vi "Read INI file.vi"(8 "error in (no error)":errorcluster, 11 "App Cluster in":T1) -> (0 "error out":errorcluster, 3 "App Cluster out":T1)   [LabVIEW 2018]
uses:
  type defs/App Cluster.ctl
  <vilib>/Utility/config.llb/Read Key (String).vi
  <vilib>/Utility/config.llb/Read Key (Double).vi
  <vilib>/Utility/config.llb/NI_LVConfig.lvlib
panel:
  out "Parameters":dbl[](array[numeric])
  out "HW":string[](array[string])
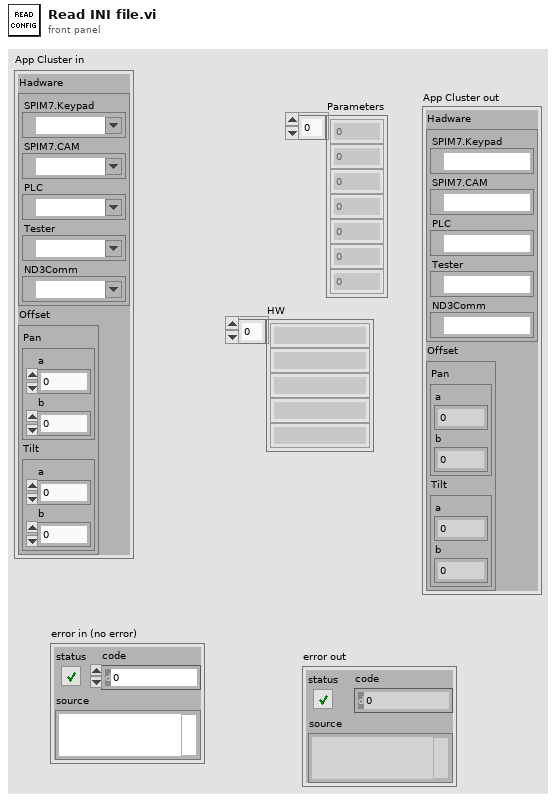
[diagram p1: front panel]
types:
  T1 = typedef "App Cluster.ctl" = cluster{"Hadware":cluster{"SPIM7.Keypad":refnum<visa-resource-name>, "SPIM7.CAM":refnum<visa-resource-name>, "PLC":refnum<visa-resource-name>, "Tester":refnum<visa-resource-name>, "ND3Comm":refnum<visa-resource-name>}, "Offset":cluster{"Pan":cluster{"a":dbl, "b":dbl}, "Tilt":cluster{"a":dbl, "b":dbl}}}
  T2 = typedef "NI_LVConfig.lvlib/Config Data RefNum.ctl" = refnum<k1>
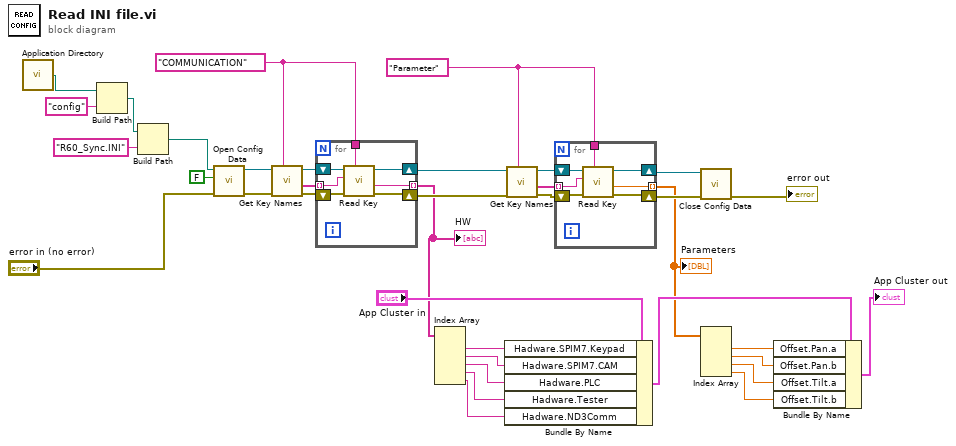
[diagram p0: block diagram]
diagram:
  w19 = "Parameter"
  w30 = "COMMUNICATION" ("section")
  n1 = call <vilib>:"Application Directory.vi"() -> ("Application Directory"=w36:path)
  n2 = Build Path(base path=w36, name or relative path="config") -> (appended path=w34:path)
  n3 = Build Path(base path=w34, name or relative path="R60_Sync.INI") -> (appended path=w32:path)
  n4 = call <vilib>:"Open Config Data.vi"("error in (no error)"="error in (no error)", "create file if necessary (T)"=FALSE, "configuration file path"=w32) -> ("error out"=w25:errorcluster, "refnum"=w29:T2)  [unwired: 6 in, 1 out]
  n5 = call <vilib>:"Get Key Names.vi"("section"=w30, "error in (no error)"=w25, "refnum"=w29) -> ("error out"=w26:errorcluster, "key names"=w27:string[], "refnum out"=w28:T2)  [unwired: 5 in, 1 out]
  n6 = for {
    tunnel: w30 -> [w43]
    tunnel: w27 -> [w41] mode=indexing
    tunnel: [w40] -> w13 mode=indexing
    shift-right: [w39] -> w23
    shift-left: w28 -> [w42]
    shift-right: [w37] -> w24
    shift-left: w26 -> [w38]
    n7 = call-poly <vilib>:"Read Key.vi"("section"=w43, "error in (no error)"=w38, "key"=w41, "refnum"=w42) -> ("error out"=w37:errorcluster, "value"=w40:string, "refnum out"=w39:T2)  [unwired: 4 in, 1 out]
  }
  "HW" <- w13
  n8 = Index Array(array=w13) -> (element #1=w11:string, element #2=w12:string, element #3=w10:string, element #4=w9:string, element #5=w8:string)  [unwired: 5 in]
  n9 = Bundle By Name(cluster="App Cluster in", "Hadware.SPIM7.Keypad"=w11, "Hadware.SPIM7.CAM"=w12, "Hadware.PLC"=w10, "Hadware.Tester"=w9, "Hadware.ND3Comm"=w8) -> (w7:T1)
  n10 = call <vilib>:"Get Key Names.vi"("section"=w19, "error in (no error)"=w24, "refnum"=w23) -> ("error out"=w21:errorcluster, "key names"=w20:string[], "refnum out"=w22:T2)  [unwired: 5 in, 1 out]
  n11 = for {
    tunnel: w19 -> [w50]
    tunnel: w20 -> [w48] mode=indexing
    tunnel: [w47] -> w6 mode=indexing
    shift-right: [w46] -> w17
    shift-left: w22 -> [w49]
    shift-right: [w44] -> w18
    shift-left: w21 -> [w45]
    n12 = call-poly <vilib>:"Read Key.vi"("section"=w50, "error in (no error)"=w45, "key"=w48, "refnum"=w49) -> ("error out"=w44:errorcluster, "value"=w47:dbl, "refnum out"=w46:T2)  [unwired: 4 in, 1 out]
  }
  "Parameters" <- w6
  n13 = call <vilib>:"Close Config Data.vi"("error in (no error)"=w18, "refnum"=w17) -> ("error out"=→"error out":errorcluster)  [unwired: 8 in, 1 out]
  n14 = Index Array(array=w6) -> (element #1=w5:dbl, element #2=w4:dbl, element #3=w3:dbl, element #4=w2:dbl)  [unwired: 4 in]
  n15 = Bundle By Name(cluster=w7, "Offset.Pan.a"=w5, "Offset.Pan.b"=w4, "Offset.Tilt.a"=w3, "Offset.Tilt.b"=w2) -> (→"App Cluster out":T1)
